vi "Log Event.vi"(8 "error in (no error)":errorcluster, 10 "value":dbl, 11 "code":dbl) -> (0 "error out":errorcluster)   [LabVIEW 2017]
uses:
  PushTask Globals.vi
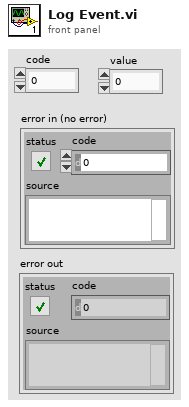
[diagram p1: front panel]
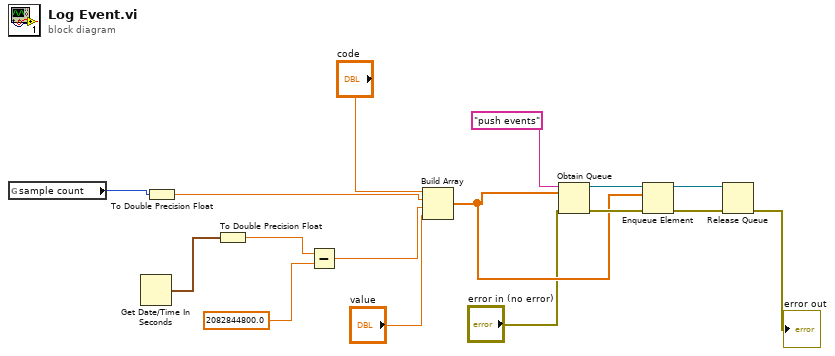
[diagram p0: block diagram]
diagram:
  n1 = global read "PushTask Globals.vi" "sample count"() -> (w15:i32)
  n2 = Get Date/Time In Seconds() -> (seconds since 1Jan1904=w16:timestamp)
  n3 = To Double Precision Float(number=w15) -> (double precision float=w11:dbl)
  n4 = To Double Precision Float(number=w16) -> (double precision float=w14:dbl)
  n5 = Subtract(x=w14, y=2082844800.0) -> (x-y=w10:dbl)
  n6 = Build Array("code", w11, w10, "value") -> (w5:dbl[])
  n7 = Obtain Queue(name (unnamed)="push events", element data type=w5, error in (no error)="error in (no error)") -> (queue out=w7:refnum<queue>, error out=w6:errorcluster)  [unwired: 2 in, 1 out]
  n8 = Enqueue Element(queue=w7, element=w5, error in (no error)=w6) -> (queue out=w4:refnum<queue>, error out=w3:errorcluster)  [unwired: 1 in, 1 out]
  n9 = Release Queue(queue=w4, error in (no error)=w3) -> (error out=→"error out":errorcluster)  [unwired: 1 in, 2 out]
